vi "Receive Messages.vi"(8 "error in":errorcluster, 10 "Sender":string, 11 "PCAN Basic Read-Write CAN Frame Strategy in":refnum<class "PCAN Basic Read-Write CAN Frame Strategy.lvclass">) -> (0 "error out":errorcluster, 2 "Messages":refnum<class "IMessage.lvclass">[](array[class]), 3 "PCAN Basic Read-Write CAN Frame Strategy out":refnum<class "PCAN Basic Read-Write CAN Frame Strategy.lvclass">)   [LabVIEW 2025, in "PCAN Basic Read-Write CAN Frame Strategy.lvclass"]
uses:
  PCAN Basic Read-Write CAN Frame Strategy.lvclass
  Source/Interfaces/IMessage/IMessage.lvclass
  Base Configure Strategy/PCAN Basic Base Configure Strategy.lvclass/PCAN Basic Base Configure Strategy.ctl
  Source/Messages/CAN Message/CAN Message.lvclass
  Source/Messages/CAN Message/CAN Message.lvclass/CAN Message.ctl
  Source/Messages/CAN Message/Set Frame Type.vi
  Base Configure Strategy/PCAN Basic Base Configure Strategy.lvclass
  <instrlib>/Peter/PCAN Basic/PCANBasic.lvlib
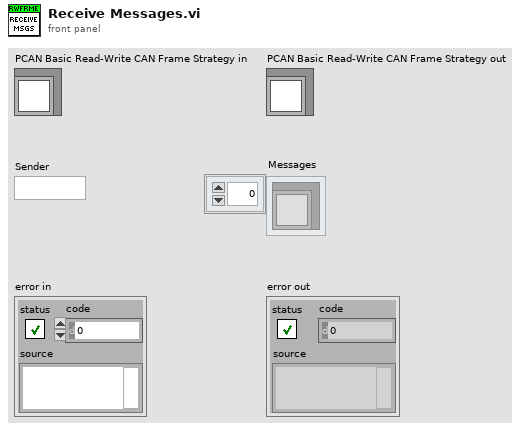
[diagram p1: front panel]
types:
  T1 = typedef "PCANBasic.lvlib/TPCANHandle.ctl" = u16
  T2 = typedef "PCANBasic.lvlib/PCAN Message.ctl" = cluster{"ID":u32, "MSGTYPE":T3, "LEN":u8, "DATA":cluster{"0":u8, "1":u8, "2":u8, "3":u8, "4":u8, "5":u8, "6":u8, "7":u8}}
  T3 = typedef "PCANBasic.lvlib/PCAN Message types.ctl" = u8
  T4 = cluster{"0":u8, "1":u8, "2":u8, "3":u8, "4":u8, "5":u8, "6":u8, "7":u8}
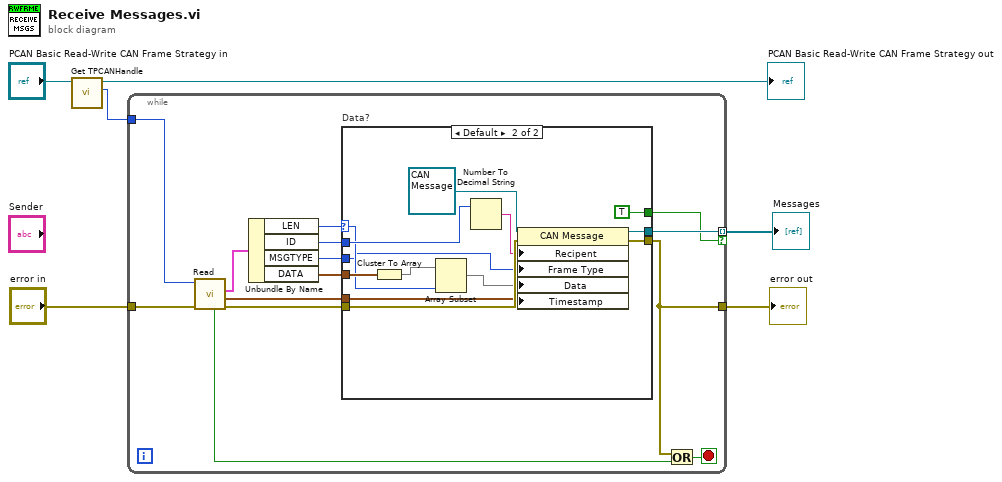
[diagram p0: block diagram]
diagram:
  n1 = call "Get TPCANHandle.vi"("PCAN Basic Base Configure Strategy in"="PCAN Basic Read-Write CAN Frame Strategy in") -> ("TPCANHandle"=w4:T1, "PCAN Basic Base Configure Strategy out"=→"PCAN Basic Read-Write CAN Frame Strategy out":refnum<class "PCAN Basic Read-Write CAN Frame Strategy.lvclass">)  [unwired: 9 in]
  n2 = while {
    tunnel: w4 -> [w20]
    tunnel: "error in" -> [w19]
    tunnel: [w7] -> w2
    tunnel: [w11] -> w1 mode=indexing if=w10
    stop <- w9 stop-if-true
    n3 = call <instrlib>:"Read.vi"("error in"=w19, "TPCANHandle in"=w20) -> ("error out"=w18:errorcluster, "Time Stamp"=w16:timestamp, "PCAN Message"=w15:T2, "Receive Queue empty"=w8:bool)  [unwired: 4 in, 2 out]
    n4 = Unbundle By Name(w15) -> ("LEN"=w17:u8, "ID"=w14:u32, "MSGTYPE"=w13:T3, "DATA"=w12:T4)
    n5 = case "Data?" shown="Default" w17 {
      selector: w17 -> [_ w25]
      tunnel: [_ w33] -> w11
      tunnel: w18 -> [w21 w32]
      tunnel: [w21 w31] -> w7
      tunnel: [_ TRUE] -> w10
      tunnel: w16 -> [_ w29]
      tunnel: w14 -> [_ w28]
      tunnel: w13 -> [_ w23]
      tunnel: w12 -> [_ w27]
      frame 0 {
      }
      frame Default {
        n6 = Cluster To Array(cluster=w27) -> (array=w26:u8[])
        n7 = Array Subset(array=w26, length=w25) -> (w24:u8[])  [unwired: 1 in]
        n8 = Number To Decimal String(number=w28) -> (decimal integer string=w30:string)  [unwired: 1 in]
        n9 = property class="CAN Message"(reference=refnum<class "CAN Message.lvclass"> refnum ("CAN Message"), error in=w32, "Recipent"=w30, "Frame Type"=w23, "Data"=w24, "Timestamp"=w29) -> (reference out=w33:refnum<class "CAN Message.lvclass">, error out=w31:errorcluster)
      }
    }
    n10 = Or(x=w7, y=w8) -> (x .or. y?=w9:bool)
  }
  "error out" <- w2
  "Messages" <- w1
